vi "Describe Write Error.vi"(7 "Config File Path":path=path "C:/ProgramData/PVI Systems/Staple Inspection System/Config.ini", 8 "error in (no error)":errorcluster, 11 "Mode":T1) -> (0 "error out":errorcluster)   [LabVIEW 2021, in "Config Module.lvlib"]
uses:
  Config Module.lvlib
  Controls/Config File Operation Enum.ctl
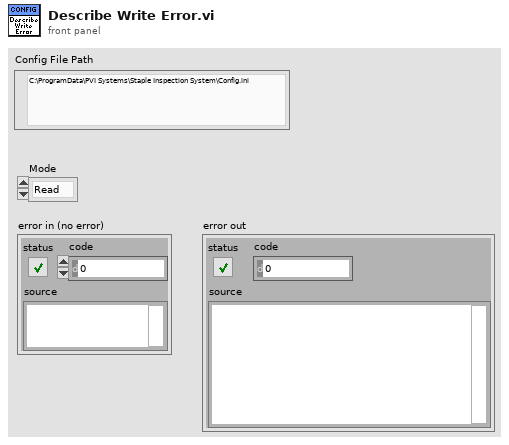
[diagram p1: front panel]
types:
  T1 = typedef "Config Module.lvlib/Config File Operation Enum.ctl" = enum16{"Read", "Write"}
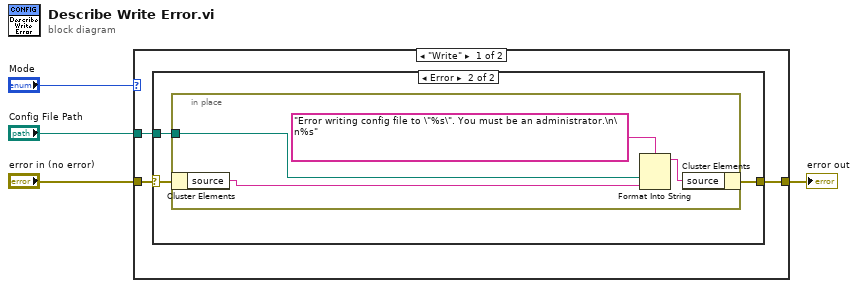
[diagram p0: block diagram]
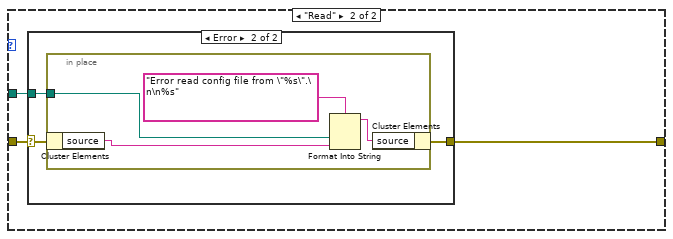
[diagram p3: hidden frame]
diagram:
  n1 = case shown="\"Write\"" "Mode" {
    tunnel: "error in (no error)" -> [w7 w18]
    tunnel: [w6 w17] -> w3
    tunnel: "Config File Path" -> [w5 w16]
    frame "Write" {
      n2 = case shown="Error" w7 {
        selector: w7 -> [w8 w10]
        tunnel: [w8 w9] -> w6
        tunnel: w5 -> [_ w11]
        frame No Error {
        }
        frame Error {
          n3 = in-place {
            in-place-border: w11 -> [w14]
            n4 = in-place-cluster #1(w10) -> ("source"=w13:string)
            n5 = Format Into String(format string="Error writing config file to \"%s\". You must be an administrator.\n\n%s", w14, w13) -> (resulting string=w12:string)  [unwired: 2 in, 1 out]
            n6 = in-place-cluster #1("source"=w12) -> (w9:errorcluster)
          }
        }
      }
    }
    frame "Read" {
      n7 = case shown="Error" w18 {
        selector: w18 -> [w19 w21]
        tunnel: [w19 w20] -> w17
        tunnel: w16 -> [_ w22]
        frame No Error {
        }
        frame Error {
          n8 = in-place {
            in-place-border: w22 -> [w25]
            n9 = in-place-cluster #2(w21) -> ("source"=w24:string)
            n10 = Format Into String(format string="Error read config file from \"%s\".\n\n%s", w25, w24) -> (resulting string=w23:string)  [unwired: 2 in, 1 out]
            n11 = in-place-cluster #2("source"=w23) -> (w20:errorcluster)
          }
        }
      }
    }
  }
  "error out" <- w3
